vi "Read4040.vi"(8 "错误输入（无错误）":errorcluster, 11 "VISA引用句柄输入":refnum<visa-resource-name>) -> (0 "错误输出":errorcluster, 2 "read buffer":string, 3 "VISA引用句柄输出":refnum<visa-resource-name>)   [LabVIEW 2017]
uses:
  <vilib>/Instr/_visa.llb/VISA Flush IO Buffer Mask.ctl
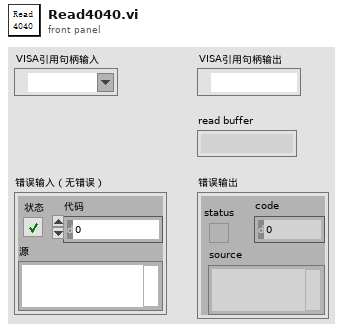
[diagram p1: front panel]
types:
  T1 = typedef "VISA Flush IO Buffer Mask.ctl" = u16
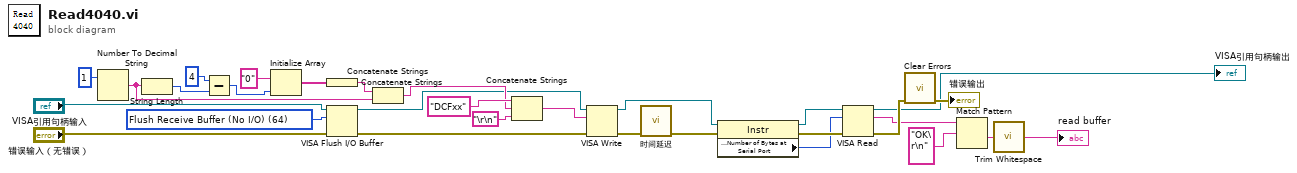
[diagram p0: block diagram]
diagram:
  w23 = T1 64 items=["Flush Receive Buffer"=16, "Write Transmit Buffer to Device"=32, "Flush Receive Buffer (No I/O)"=64, "Flush Transmit Buffer"=128] ("Mask")
  n1 = Number To Decimal String(number=1 ("sample number")) -> (decimal integer string=w13:string)  [unwired: 1 in]
  n2 = String Length(string=w13) -> (length=w9:i32)
  n3 = Subtract(x=4, y=w9) -> (x-y=w10:i32)
  n4 = Initialize Array("0", w10) -> (w11:string[])
  n5 = Concatenate Strings(w11) -> (w12:string)
  n6 = VISA Flush I/O Buffer(VISA resource name="VISA引用句柄输入", mask (16)=w23, error in (no error)="错误输入（无错误）") -> (VISA resource name out=w6:refnum<visa-resource-name>, error out=w18:errorcluster)
  n7 = Concatenate Strings(w12, w13) -> (w14:string)
  n8 = Concatenate Strings("DCFxx" ("写入缓冲区"), w14, "\r\n") -> (w15:string)
  n9 = VISA Write(VISA resource name=w6, write buffer=w15, error in (no error)=w18) -> (VISA resource name out=w3:refnum<visa-resource-name>, error out=w8:errorcluster)  [unwired: 1 out]
  n10 = call "时间延迟"("error in (no error)"=w8) -> ("error out"=w7:errorcluster)  [unwired: 10 in]
  n11 = property class="Instr"(reference=w3, error in=w7) -> (reference out=w2:refnum<visa-resource-name>, error out=w4:errorcluster, "Serial Settings:Number of Bytes at Serial Port"=w1:u32)
  n12 = VISA Read(VISA resource name=w2, byte count=w1, error in (no error)=w4) -> (VISA resource name out=→"VISA引用句柄输出":refnum<visa-resource-name>, read buffer=w16:string, error out=w30:errorcluster)  [unwired: 1 out]
  n13 = call <vilib>:"Clear Errors.vi"("error in (no error)"=w30) -> ("error out"=→"错误输出":errorcluster)  [unwired: 5 in, 1 out]
  n14 = Match Pattern(string=w16, regular expression="OK\r\n" ("正则表达式")) -> (after substring=w17:string)  [unwired: 1 in, 3 out]
  n15 = call <vilib>:"Trim Whitespace.vi"("string"=w17) -> ("trimmed string"=→"read buffer":string)  [unwired: 1 in]
